vi "MAAP2.vi"() -> ()   [LabVIEW 2016]
doc: "The VI loads the data from a file and perform an eyeball fit to the data. User can save the normalized and fitting data in a spreadsheet.\n\nMuhannad Alghamdi\nProject 2\nPhysics 350"
uses:
  typedefs/fitting_parameters_for_ke.ctl
panel:
  out "Data read":dbl[][](array[numeric]) format="%#_3g"
  in  "Save data":bool
  out "Output data":dbl[][](array[numeric]) format="%#_3g"
  out "Normalized kinetic energy":cluster{i32[], "y fit array":dbl[]}[](graph)
  in  "Fitting parameters":T1={"A"=1.6, "B"=0.001, "C"=2200.0, "D"=-0.2} {"D" scale=-1.0..1.0; "C" scale=0.0..3000.0; "B" scale=0.0..0.002; "A" scale=0.0..2.0}
  in  "Stop":bool
  out "Kinetic energy":dbl[](graph)
  out "Position":dbl[](graph)
  out "Size":i32[](array[numeric])=[2, 10000]
  out "Header string":string="position of an individual particle\nand kinetic energy of both \nfor a two LJ particle system decaying to zero due to artificial drag\n\nproduced by LJ simulation (P350, exercise 4)\n\n1/25/17\n"
  # "Lennard Jones Energy Simulation Data (Golden Version)"
  # "Muhannad Alghamdi\nProject 2\nPhysics 350"
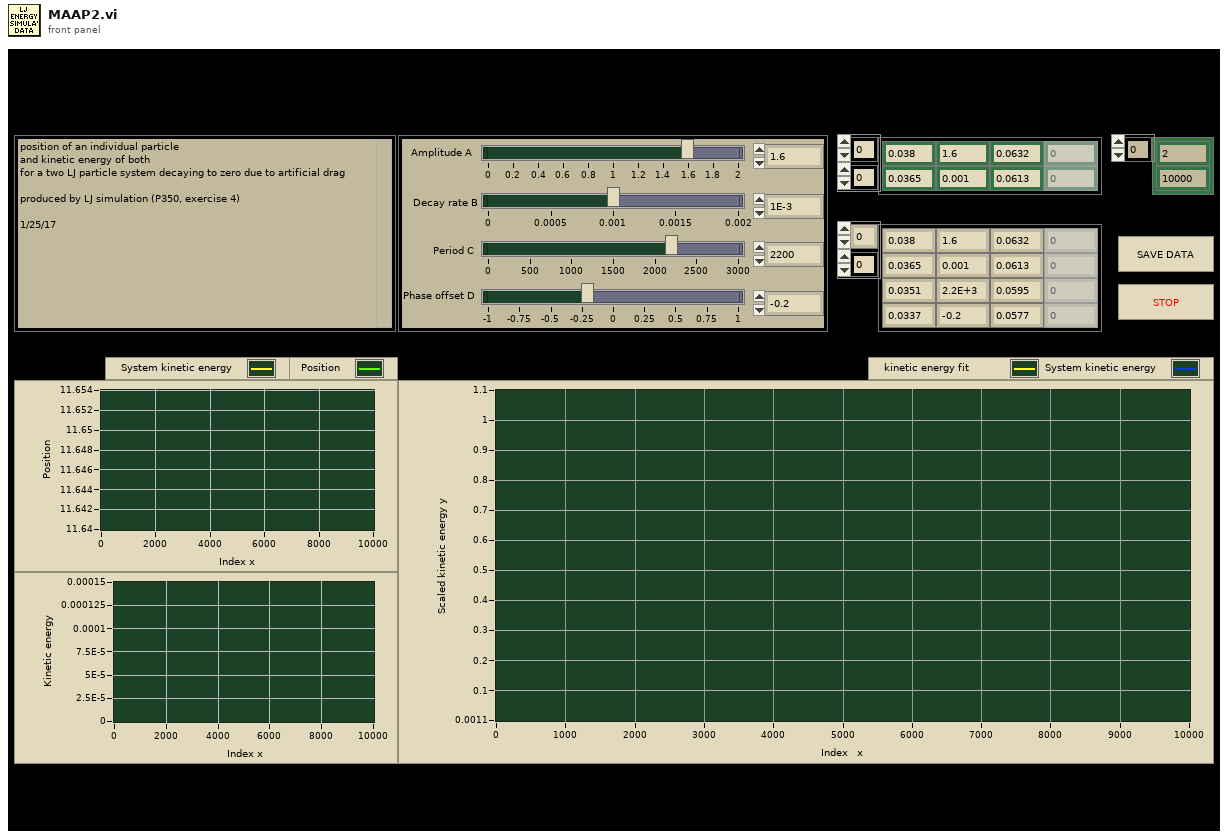
[diagram p1: front panel]
types:
  T1 = typedef "fitting_parameters_for_ke.ctl" = cluster{"A":dbl, "B":dbl, "C":dbl, "D":dbl}
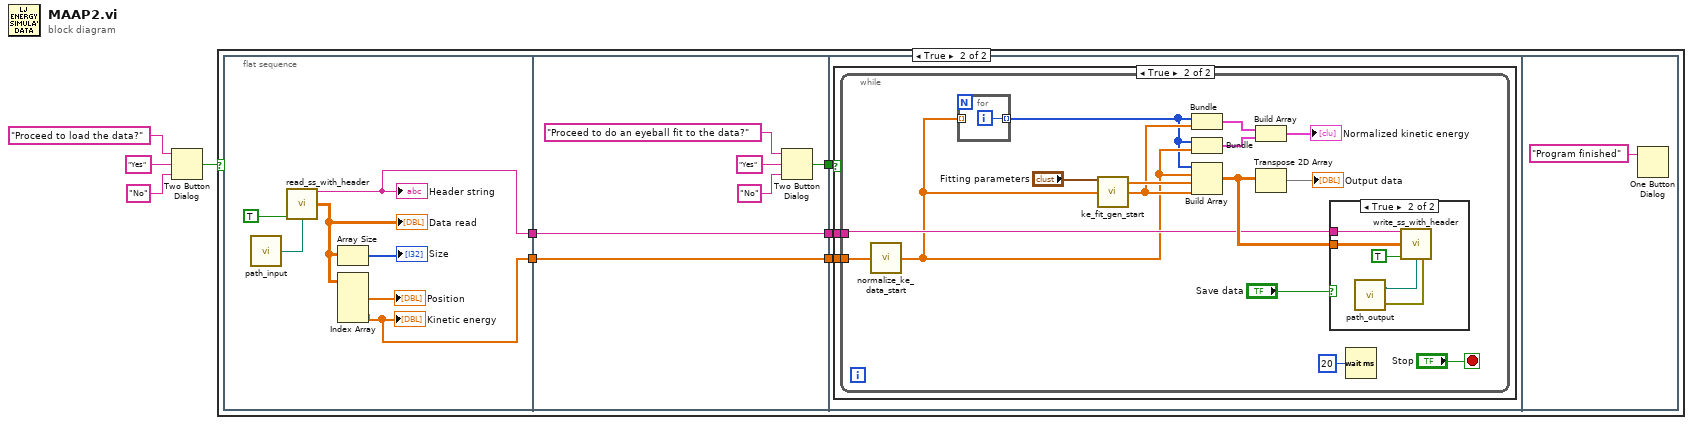
[diagram p0: block diagram]
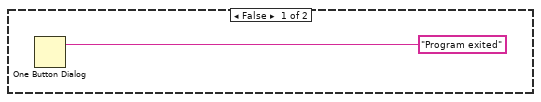
[diagram p2: hidden frame]
diagram:
  n1 = Two Button Dialog(message="Proceed to load the data?", 1:"No" ("F button name (\"Cancel\")"), 2:"Yes" ("T button name (\"OK\")")) -> (T button?=w4:bool)
  n2 = case shown="True" w4 {
    frame False {
      n3 = One Button Dialog(message="Program exited") -> ()  [unwired: 1 in, 1 out]
    }
    frame True {
      n4 = flat-sequence {
        tunnel: [w13] -> w8
        tunnel: [w14] -> w6
        tunnel: [w20] -> w10
        tunnel: [w19] -> w9
        tunnel: w8 -> [w19]
        tunnel: [w18] -> w7
        tunnel: w6 -> [w18]
        tunnel: w10 -> [w26]
        tunnel: w9 -> [w25]
        tunnel: w7 -> [w24]
        frame #0 {
          n5 = call "path_input.vi"() -> ("Path input"=w11:path)  [unwired: 1 in]
          n6 = call "read_ss_with_header.vi"("Transpose Data Array"=TRUE, "file (use dialog)"=w11) -> ("Header String"=w13:string, "Data Read"=w12:dbl[][])  [unwired: 11 in, 1 out]
          "Header string" <- w13
          "Data read" <- w12
          n7 = Array Size(array=w12) -> (size(s)=→"Size":i32[])
          n8 = Index Array(array=w12) -> (element #1=→"Position":dbl[], element #2=w14:dbl[])  [unwired: 4 in]
          "Kinetic energy" <- w14
        }
        frame #1 {
          n9 = Two Button Dialog(message="Proceed to do an eyeball fit to the data?", 1:"No" ("F button name (\"Cancel\")"), 2:"Yes" ("T button name (\"OK\")")) -> (T button?=w20:bool)
        }
        frame #2 {
          n10 = case shown="True" w26 {
            tunnel: w25 -> [_ w28]
            tunnel: w24 -> [_ w27]
            frame False {
            }
            frame True {
              n11 = while {
                tunnel: w28 -> [w32]
                tunnel: w27 -> [w33]
                stop <- "Stop" stop-if-true
                n12 = call "normalize_ke_data_start.vi"("Raw y data"=w33) -> ("Normalized y data"=w31:dbl[])  [unwired: 14 in]
                n13 = for {
                  tunnel: [w49] -> w30 mode=indexing
                  tunnel: w31 -> [_] mode=indexing
                  i -> [w49]
                }
                n14 = call "ke_fit_gen_start.vi"("Fitting parameters"="Fitting parameters", "x array"=w31) -> ("Fitting paramters array"=w37:dbl[], "y fit array"=w36:dbl[])  [unwired: 12 in]
                n15 = Bundle(w30, "y fit array"=w36) -> (w41:cluster{i32[], "y fit array":dbl[]})  [unwired: 1 in]
                n16 = Bundle(w30, "Normalized y data"=w31) -> (w40:cluster{i32[], "Normalized y data":dbl[]})  [unwired: 1 in]
                n17 = Build Array(w30, w31, w37, w36) -> (w34:dbl[][])
                n18 = Build Array(w41, w40) -> (→"Normalized kinetic energy":cluster{i32[], "Normalized y data":dbl[]}[])
                n19 = Transpose 2D Array(2D array=w34) -> (transposed array=→"Output data":dbl[][])
                n20 = case shown="True" "Save data" {
                  tunnel: w34 -> [_ w48]
                  tunnel: w32 -> [_ w46]
                  frame False {
                  }
                  frame True {
                    n21 = call "path_output.vi"() -> ("Path output"=w45:path, "Error out"=w44:errorcluster)  [unwired: 1 in]
                    n22 = call "write_ss_with_header.vi"("Header String"=w46, "Data to Write"=w48, "Transpose Data?"=TRUE, "file (use dialog)"=w45, "Error in"=w44) -> ()  [unwired: 11 in]
                  }
                }
                n23 = Wait (ms)(milliseconds to wait=u32 20) -> ()  [unwired: 1 out]
              }
            }
          }
        }
        frame #3 {
          n24 = One Button Dialog(message="Program finished") -> ()  [unwired: 1 in, 1 out]
        }
      }
    }
  }
